vi "校准信息解析.vi"(11 "校准信息":u16[](array[numeric]) caption="关键参数") -> ()   [LabVIEW 2016, in "数据传输系统.lvlib"]
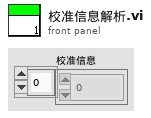
[diagram p1: front panel]
types:
  T1 = cluster{"低标液1浓度":dbl, "低标液1信号值":dbl, "低标液1启用":u16, "低标液2浓度":dbl, "低标液2信号值":dbl, "低标液2启用":u16, "低标液3浓度":dbl, "低标液3信号值":dbl, "低标液3启用":u16, "低标液4浓度":dbl, "低标液4信号值":dbl, "低标液4启用":u16, "低标液5浓度":dbl, "低标液5信号值":dbl, "低标液5启用":u16, "高标液1浓度":dbl, "高标液1信号值":dbl, "高标液1启用":u16, "高标液2浓度":dbl, "高标液2信号值":dbl, "高标液2启用":u16, "高标液3浓度":dbl, "高标液3信号值":dbl, "高标液3启用":u16, "高标液4浓度":dbl, "高标液4信号值":dbl, "高标液4启用":u16, "高标液5浓度":dbl, "高标液5信号值":dbl, "高标液5启用":u16}
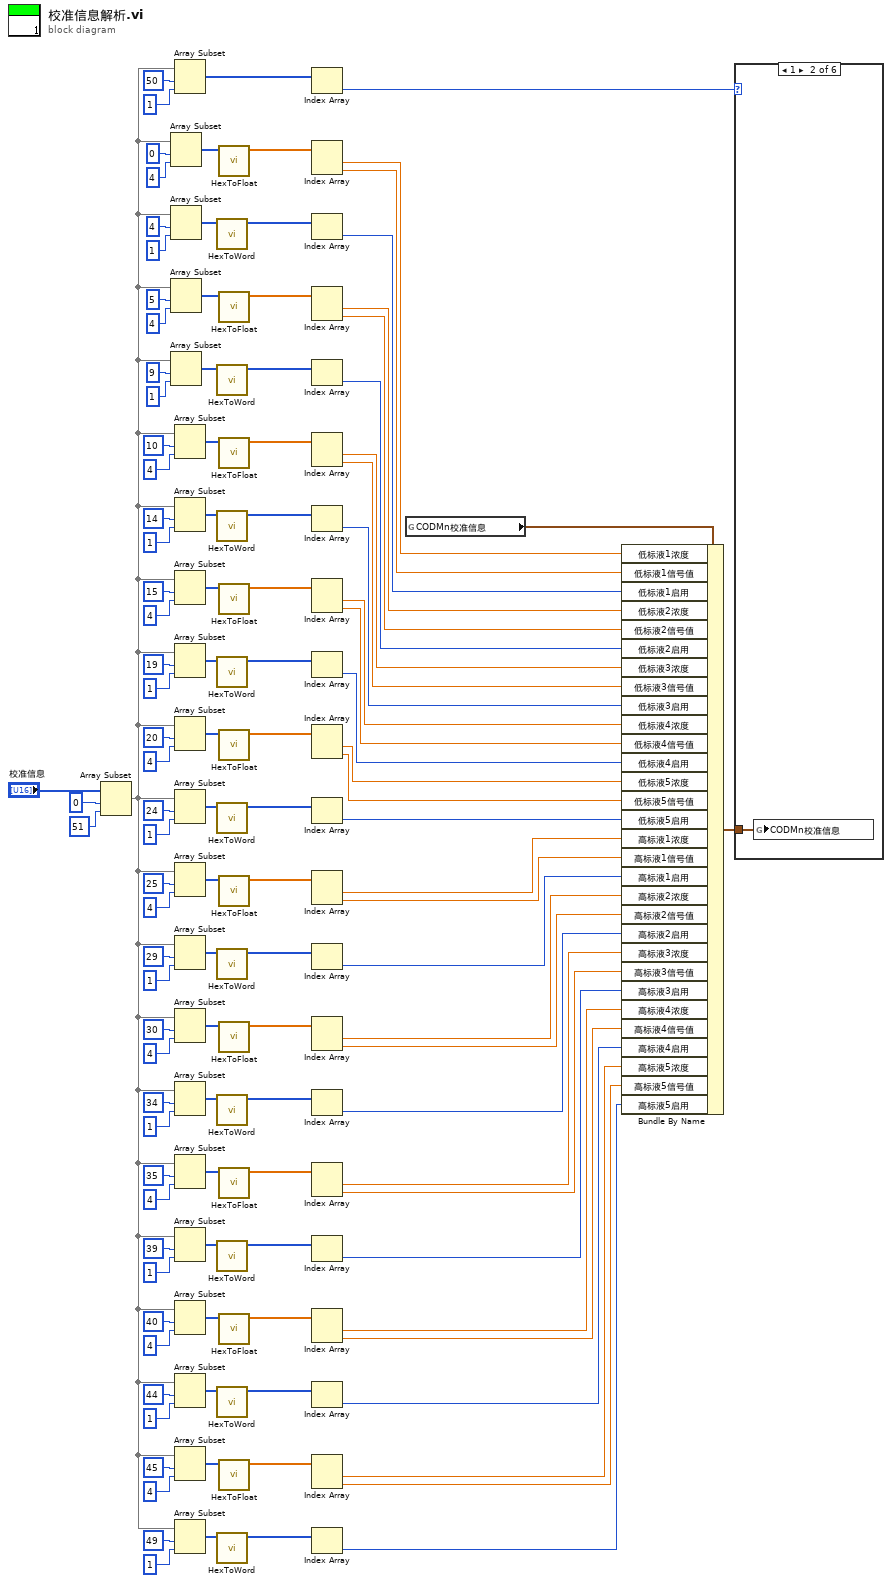
[diagram p0: block diagram]
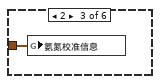
[diagram p3: hidden frame]
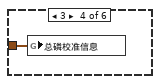
[diagram p4: hidden frame]
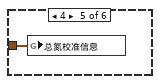
[diagram p5: hidden frame]
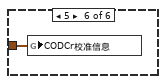
[diagram p6: hidden frame]
diagram:
  n1 = Array Subset(array="校准信息", index=0 ("y"), length=51 ("长度")) -> (w5:u16[])
  n2 = Array Subset(array=w5, index=0 ("索引"), length=4 ("长度")) -> (w114:u16[])
  n3 = Array Subset(array=w5, index=4 ("索引"), length=1 ("长度")) -> (w104:u16[])
  n4 = Array Subset(array=w5, index=5 ("索引"), length=4 ("长度")) -> (w53:u16[])
  n5 = Array Subset(array=w5, index=9 ("索引"), length=1 ("长度")) -> (w54:u16[])
  n6 = Array Subset(array=w5, index=50 ("索引"), length=1 ("长度")) -> (w1:u16[])
  n7 = Array Subset(array=w5, index=10 ("索引"), length=4 ("长度")) -> (w49:u16[])
  n8 = Array Subset(array=w5, index=14 ("索引"), length=1 ("长度")) -> (w48:u16[])
  n9 = Array Subset(array=w5, index=15 ("索引"), length=4 ("长度")) -> (w44:u16[])
  n10 = Array Subset(array=w5, index=19 ("索引"), length=1 ("长度")) -> (w42:u16[])
  n11 = Array Subset(array=w5, index=20 ("索引"), length=4 ("长度")) -> (w35:u16[])
  n12 = Array Subset(array=w5, index=24 ("索引"), length=1 ("长度")) -> (w34:u16[])
  n13 = Array Subset(array=w5, index=25 ("索引"), length=4 ("长度")) -> (w33:u16[])
  n14 = Array Subset(array=w5, index=29 ("索引"), length=1 ("长度")) -> (w32:u16[])
  n15 = Array Subset(array=w5, index=30 ("索引"), length=4 ("长度")) -> (w19:u16[])
  n16 = Array Subset(array=w5, index=34 ("索引"), length=1 ("长度")) -> (w20:u16[])
  n17 = Array Subset(array=w5, index=35 ("索引"), length=4 ("长度")) -> (w16:u16[])
  n18 = Array Subset(array=w5, index=39 ("索引"), length=1 ("长度")) -> (w15:u16[])
  n19 = Array Subset(array=w5, index=40 ("索引"), length=4 ("长度")) -> (w12:u16[])
  n20 = Array Subset(array=w5, index=44 ("索引"), length=1 ("长度")) -> (w11:u16[])
  n21 = Array Subset(array=w5, index=45 ("索引"), length=4 ("长度")) -> (w6:u16[])
  n22 = Array Subset(array=w5, index=49 ("索引"), length=1 ("长度")) -> (w4:u16[])
  n23 = call "HexToWord.vi"("数组"=w104) -> ("WORD"=w103:u16[])  [unwired: 10 in]
  n24 = call "HexToWord.vi"("数组"=w54) -> ("WORD"=w101:u16[])  [unwired: 10 in]
  n25 = call "HexToWord.vi"("数组"=w48) -> ("WORD"=w90:u16[])  [unwired: 10 in]
  n26 = call "HexToWord.vi"("数组"=w42) -> ("WORD"=w89:u16[])  [unwired: 10 in]
  n27 = call "HexToWord.vi"("数组"=w34) -> ("WORD"=w80:u16[])  [unwired: 10 in]
  n28 = call "HexToWord.vi"("数组"=w32) -> ("WORD"=w79:u16[])  [unwired: 10 in]
  n29 = call "HexToWord.vi"("数组"=w20) -> ("WORD"=w70:u16[])  [unwired: 10 in]
  n30 = call "HexToWord.vi"("数组"=w15) -> ("WORD"=w69:u16[])  [unwired: 10 in]
  n31 = call "HexToWord.vi"("数组"=w11) -> ("WORD"=w60:u16[])  [unwired: 10 in]
  n32 = call "HexToWord.vi"("数组"=w4) -> ("WORD"=w59:u16[])  [unwired: 10 in]
  n33 = call "HexToFloat.vi"("数组"=w114) -> ("FLOAT"=w113:sgl[])  [unwired: 10 in]
  n34 = call "HexToFloat.vi"("数组"=w53) -> ("FLOAT"=w100:sgl[])  [unwired: 10 in]
  n35 = call "HexToFloat.vi"("数组"=w49) -> ("FLOAT"=w91:sgl[])  [unwired: 10 in]
  n36 = call "HexToFloat.vi"("数组"=w44) -> ("FLOAT"=w88:sgl[])  [unwired: 10 in]
  n37 = call "HexToFloat.vi"("数组"=w35) -> ("FLOAT"=w81:sgl[])  [unwired: 10 in]
  n38 = call "HexToFloat.vi"("数组"=w33) -> ("FLOAT"=w78:sgl[])  [unwired: 10 in]
  n39 = call "HexToFloat.vi"("数组"=w19) -> ("FLOAT"=w71:sgl[])  [unwired: 10 in]
  n40 = call "HexToFloat.vi"("数组"=w16) -> ("FLOAT"=w68:sgl[])  [unwired: 10 in]
  n41 = call "HexToFloat.vi"("数组"=w12) -> ("FLOAT"=w61:sgl[])  [unwired: 10 in]
  n42 = call "HexToFloat.vi"("数组"=w6) -> ("FLOAT"=w58:sgl[])  [unwired: 10 in]
  n43 = Index Array(array=w1) -> (element=w106:u16)  [unwired: 1 in]
  n44 = Index Array(array=w113) -> (element #1=w112:sgl, element #2=w111:sgl)  [unwired: 2 in]
  n45 = Index Array(array=w103) -> (element=w102:u16)  [unwired: 1 in]
  n46 = Index Array(array=w100) -> (element #1=w52:sgl, element #2=w51:sgl)  [unwired: 2 in]
  n47 = Index Array(array=w101) -> (element=w50:u16)  [unwired: 1 in]
  n48 = Index Array(array=w91) -> (element #1=w47:sgl, element #2=w46:sgl)  [unwired: 2 in]
  n49 = Index Array(array=w90) -> (element=w45:u16)  [unwired: 1 in]
  n50 = Index Array(array=w88) -> (element #1=w31:sgl, element #2=w30:sgl)  [unwired: 2 in]
  n51 = Index Array(array=w89) -> (element=w29:u16)  [unwired: 1 in]
  n52 = Index Array(array=w81) -> (element #1=w28:sgl, element #2=w27:sgl)  [unwired: 2 in]
  n53 = Index Array(array=w80) -> (element=w26:u16)  [unwired: 1 in]
  n54 = Index Array(array=w78) -> (element #1=w25:sgl, element #2=w24:sgl)  [unwired: 2 in]
  n55 = Index Array(array=w79) -> (element=w23:u16)  [unwired: 1 in]
  n56 = Index Array(array=w71) -> (element #1=w22:sgl, element #2=w21:sgl)  [unwired: 2 in]
  n57 = Index Array(array=w70) -> (element=w18:u16)  [unwired: 1 in]
  n58 = Index Array(array=w68) -> (element #1=w17:sgl, element #2=w14:sgl)  [unwired: 2 in]
  n59 = Index Array(array=w69) -> (element=w13:u16)  [unwired: 1 in]
  n60 = Index Array(array=w61) -> (element #1=w10:sgl, element #2=w9:sgl)  [unwired: 2 in]
  n61 = Index Array(array=w60) -> (element=w8:u16)  [unwired: 1 in]
  n62 = Index Array(array=w58) -> (element #1=w7:sgl, element #2=w3:sgl)  [unwired: 2 in]
  n63 = Index Array(array=w59) -> (element=w2:u16)  [unwired: 1 in]
  n64 = global read "全局1.vi" "CODMn校准信息"() -> (w105:T1)
  n65 = Bundle By Name(cluster=w105, "低标液1浓度"=w112, "低标液1信号值"=w111, "低标液1启用"=w102, "低标液2浓度"=w52, "低标液2信号值"=w51, "低标液2启用"=w50, "低标液3浓度"=w47, "低标液3信号值"=w46, "低标液3启用"=w45, "低标液4浓度"=w31, "低标液4信号值"=w30, "低标液4启用"=w29, "低标液5浓度"=w28, "低标液5信号值"=w27, "低标液5启用"=w26, "高标液1浓度"=w25, "高标液1信号值"=w24, "高标液1启用"=w23, "高标液2浓度"=w22, "高标液2信号值"=w21, "高标液2启用"=w18, "高标液3浓度"=w17, "高标液3信号值"=w14, "高标液3启用"=w13, "高标液4浓度"=w10, "高标液4信号值"=w9, "高标液4启用"=w8, "高标液5浓度"=w7, "高标液5信号值"=w3, "高标液5启用"=w2) -> (w119:T1)
  n66 = case shown="1" w106 {
    tunnel: w119 -> [_ w121 w122 w123 w124 w125]
    frame 0, Default {
    }
    frame 1 {
      n67 = global write "全局1.vi" "CODMn校准信息"(w121) -> ()
    }
    frame 2 {
      n68 = global write "全局1.vi" "氨氮校准信息"(w122) -> ()
    }
    frame 3 {
      n69 = global write "全局1.vi" "总磷校准信息"(w123) -> ()
    }
    frame 4 {
      n70 = global write "全局1.vi" "总氮校准信息"(w124) -> ()
    }
    frame 5 {
      n71 = global write "全局1.vi" "CODCr校准信息"(w125) -> ()
    }
  }
